vi "initializeRobots.vi"(8 "error in (no error)":errorcluster, 11 "Game in":refnum<class "Game.lvclass">) -> (0 "error out":errorcluster, 3 "Game out":refnum<class "Game.lvclass">)   [LabVIEW 2018, in "Game.lvclass"]
uses:
  Game.lvclass
  Robot_class/Robot.lvclass
  Game.lvclass/Game.ctl
  Team_class/Team.lvclass/Team.ctl
  Read AllyRef.vi
  Read EnemyRef.vi
  Team_class/Write RobotRef.vi
  Write AllyRef.vi
  Write EnemyRef.vi
  Enemy_class/Enemy.lvclass
  C:/Users/Ronaldo/Desktop/Phoenix/SSL_AI/Team_class/Team.lvclass
  Ally_class/Ally.lvclass
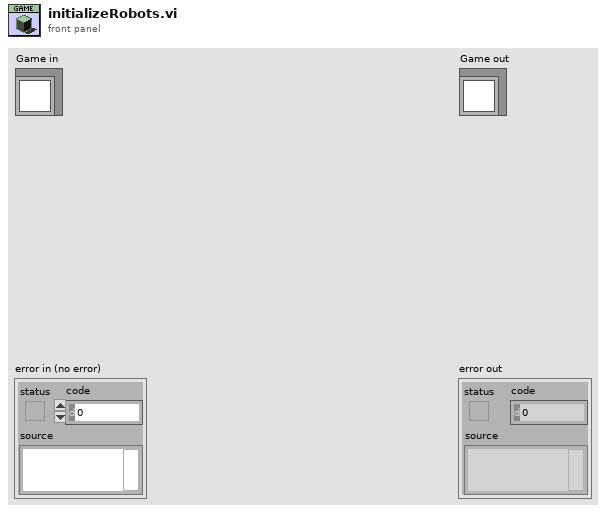
[diagram p1: front panel]
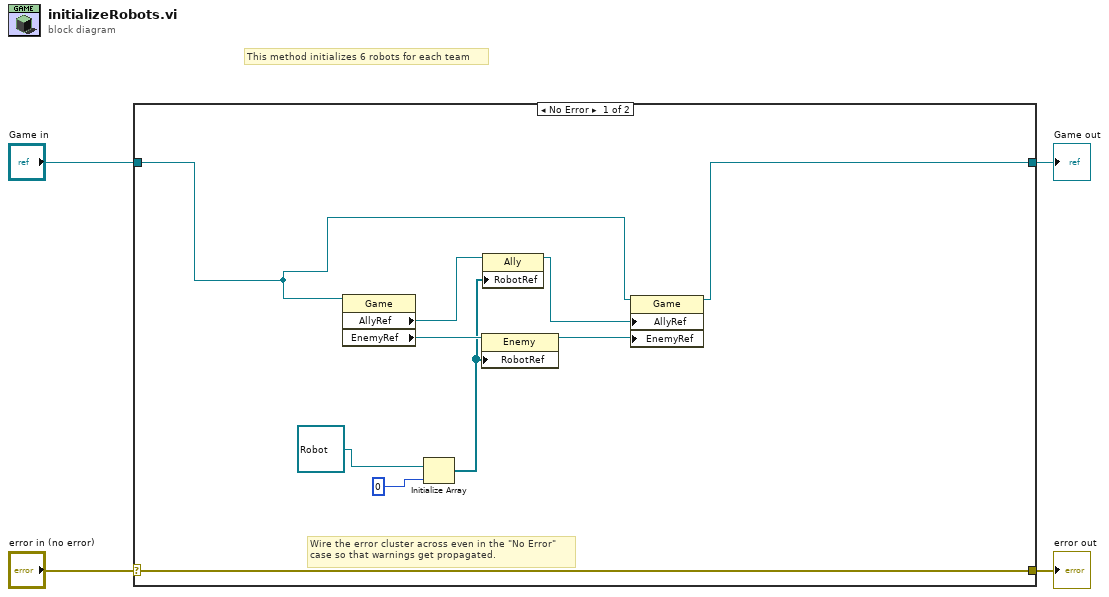
[diagram p0: block diagram]
diagram:
  # "This method initializes 6 robots for each team"
  n1 = case shown="No Error" "error in (no error)" {
    selector: "error in (no error)" -> [w14 w16]
    tunnel: [w14 w16] -> w3
    tunnel: [w5 w15] -> w1
    tunnel: "Game in" -> [w6 w15]
    frame No Error {
      # "Wire the error cluster across even in the \"No Error\"\ncase so that warnings get propagated."
      n2 = property class="Game"(reference=w6) -> ("AllyRef"=w11:refnum<class "Ally.lvclass">, "EnemyRef"=w10:refnum<class "Enemy.lvclass">)  [unwired: 1 in, 2 out]
      n3 = Initialize Array(refnum<class "Robot.lvclass"> refnum ("Robot"), 0 ("dimension size")) -> (w9:refnum<class "Robot.lvclass">[])
      n4 = property class="Enemy"(reference=w10, "RobotRef"=w9) -> (reference out=w7:refnum<class "Enemy.lvclass">)  [unwired: 1 in, 1 out]
      n5 = property class="Ally"(reference=w11, "RobotRef"=w9) -> (reference out=w8:refnum<class "Ally.lvclass">)  [unwired: 1 in, 1 out]
      n6 = property class="Game"(reference=w6, "AllyRef"=w8, "EnemyRef"=w7) -> (reference out=w5:refnum<class "Game.lvclass">)  [unwired: 1 in, 1 out]
    }
    frame Error {
    }
  }
  "error out" <- w3
  "Game out" <- w1
